vi "Configure.vi"(8 "error in (no error)":errorcluster) -> (0 "error out":errorcluster, 2 "groups":string[](array[string]), 3 "config":variant)   [LabVIEW 2017, in "DataAccumulator.lvlib"]
uses:
  <vilib>/addons/InsightCM/Devices/Shared/Common/DataAccumulator/DataAccumulator.lvlib
  <vilib>/addons/InsightCM/Devices/Shared/Common/DataAccumulator/controls/DataStoreOps.ctl
  <vilib>/addons/InsightCM/Devices/Shared/Common/DataAccumulator/controls/config.ctl
  <vilib>/addons/InsightCM/Devices/Shared/Common/DeviceHealth/controls/deviceHealthTag.ctl
  <vilib>/addons/InsightCM/Devices/Shared/Common/DeviceHealth/controls/SystemHealthTagEnum.ctl
  <vilib>/addons/InsightCM/MessageBus/Base/controls/Tag.ctl
  <vilib>/addons/InsightCM/MessageBus/Base/controls/KeyValuePair.ctl
  <vilib>/addons/InsightCM/Devices/Shared/Common/DataAccumulator/controls/AccumulationSettings.ctl
  <vilib>/addons/InsightCM/Devices/Shared/Common/DataAccumulator/controls/accumulationType.ctl
  <vilib>/addons/InsightCM/Devices/Shared/Common/DVRBuffer/controls/BufferLocation.ctl
  <vilib>/addons/InsightCM/Devices/Shared/Common/DVRBuffer/DVRBuffer.lvlib
  <vilib>/addons/InsightCM/Utilities/GlobalConfiguration/GlobalConfiguration.lvlib
  <vilib>/addons/InsightCM/Utilities/DeviceModelHelpers/DeviceModelHelpers.lvlib
  <vilib>/addons/InsightCM/Utilities/PropertyHelpers/PropertyHelpers.lvlib
  <vilib>/addons/InsightCM/Devices/Shared/Common/DeviceHealth/DeviceHealth.lvlib
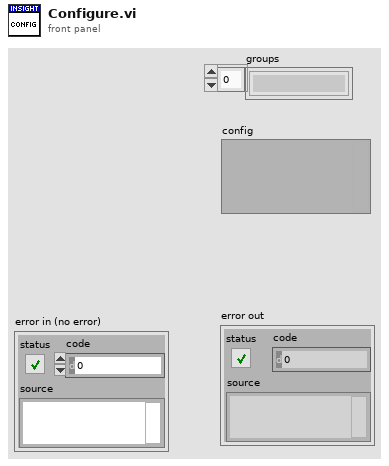
[diagram p1: front panel]
types:
  T1 = typedef "DataAccumulator.lvlib/DataStoreOps.ctl" = enum16{"Reset", "Init", "Clear", "SetWfms", "GetWfms"}
  T2 = typedef "SectionKeyValues.ctl" = cluster{"Section":string, "KeyValues":T3[]}
  T3 = typedef "KeyValuePair.ctl" = cluster{"Key":string, "Value":string}
  T4 = typedef "R2_DeviceModel.ctl" = cluster{"Device":T5, "Channels":T12[], "Tags":T14[]}
  T5 = typedef "R2_Device.ctl" = cluster{"Id":string, "Name":string, "DeviceType":string, "HardwareName":string, "IpAddress":string, "HardwareInfo":T3[], "ApplicationType":string, "ApplicationVersion":string, "EquipmentIds":string[], "ConfigurationVersion":string, "State":T6, "Properties":T3[], "DataGroups":T7[], "BurstModeTrigger":T11}
  T6 = typedef "DeviceState.ctl" = cluster{"Disabled":bool}
  T7 = typedef "R2_DataGroup.ctl" = cluster{"Name":string, "OperatingStates":T8[], "Properties":T3[], "EquipmentIds":string[], "AssetNodeId":string}
  T8 = typedef "OperatingState.ctl" = cluster{"Name":string, "Properties":T3[], "Triggers":T9[]}
  T9 = typedef "Trigger.ctl" = cluster{"Type":string, "Expression":string, "Conditions":T10[]}
  T10 = typedef "Condition.ctl" = cluster{"Source":string, "Type":string, "Operator":string, "CompareTo":string, "DwellSeconds":dbl}
  T11 = typedef "BurstModeTrigger.ctl" = cluster{"Trigger":T9, "SampleRate":string, "AcquisitionLength":string}
  T12 = typedef "R2_Channel.ctl" = cluster{"Id":string, "DeviceId":string, "Name":string, "ChannelType":string, "HardwareKey":string, "HardwareChannel":string, "DataGroup":string, "Keywords":string[], "EquipmentIds":string[], "Properties":T3[], "Metrics":T13[], "AssetNodeId":string, "MeasType":string, "AssetName":string}
  T13 = typedef "Metric.ctl" = cluster{"Id":string, "Name":string, "Unit":string, "Properties":T3[], "MetricDefinitionInstanceId":string}
  T14 = typedef "Tag.ctl" = cluster{"Id":string, "Path":string, "Name":string, "Datatype":string, "Props":T3[], "Keywords":string[]}
  T15 = typedef "DataAccumulator.lvlib/config.ctl" = cluster{"Group":string, "BlockComplete":bool, "Ok To Start":bool, "Speed Ref Chan":string, "Current OpState":string, "MaxLowRateCPU(%)":dbl, "MaxLowRateMem(%)":dbl, "LowRateCount":i32, "LowRateCountTag":T16}
  T16 = typedef "DeviceHealth.lvlib/deviceHealthTag.ctl" = cluster{"SystemTags":T17, "TagId":string, "Tag":T14}
  T17 = typedef "DeviceHealth.lvlib/SystemHealthTagEnum.ctl" = enum16{"CPU Utilization", "Memory Utilization", "Disk Utilization", "Total Physical Memory", "Primary Disk Free", "Chassis Temperature", "LowRateCount"}
  T18 = typedef "DataAccumulator.lvlib/AccumulationSettings.ctl" = cluster{"Type":T19, "Length":dbl, "Max Time (sec)":dbl, "Start Block":T20, "Acquired (sec)":dbl, "Acquired (pulses)":i32, "Initial Pulse Offset":dbl, "Stop Block":T20, "LastBlockAdded":u32}
  T19 = typedef "DataAccumulator.lvlib/accumulationType.ctl" = enum16{"none", "seconds", "revolutions"}
  T20 = typedef "DVRBuffer.lvlib/BufferLocation.ctl" = cluster{"Block":u32, "Index":i32}
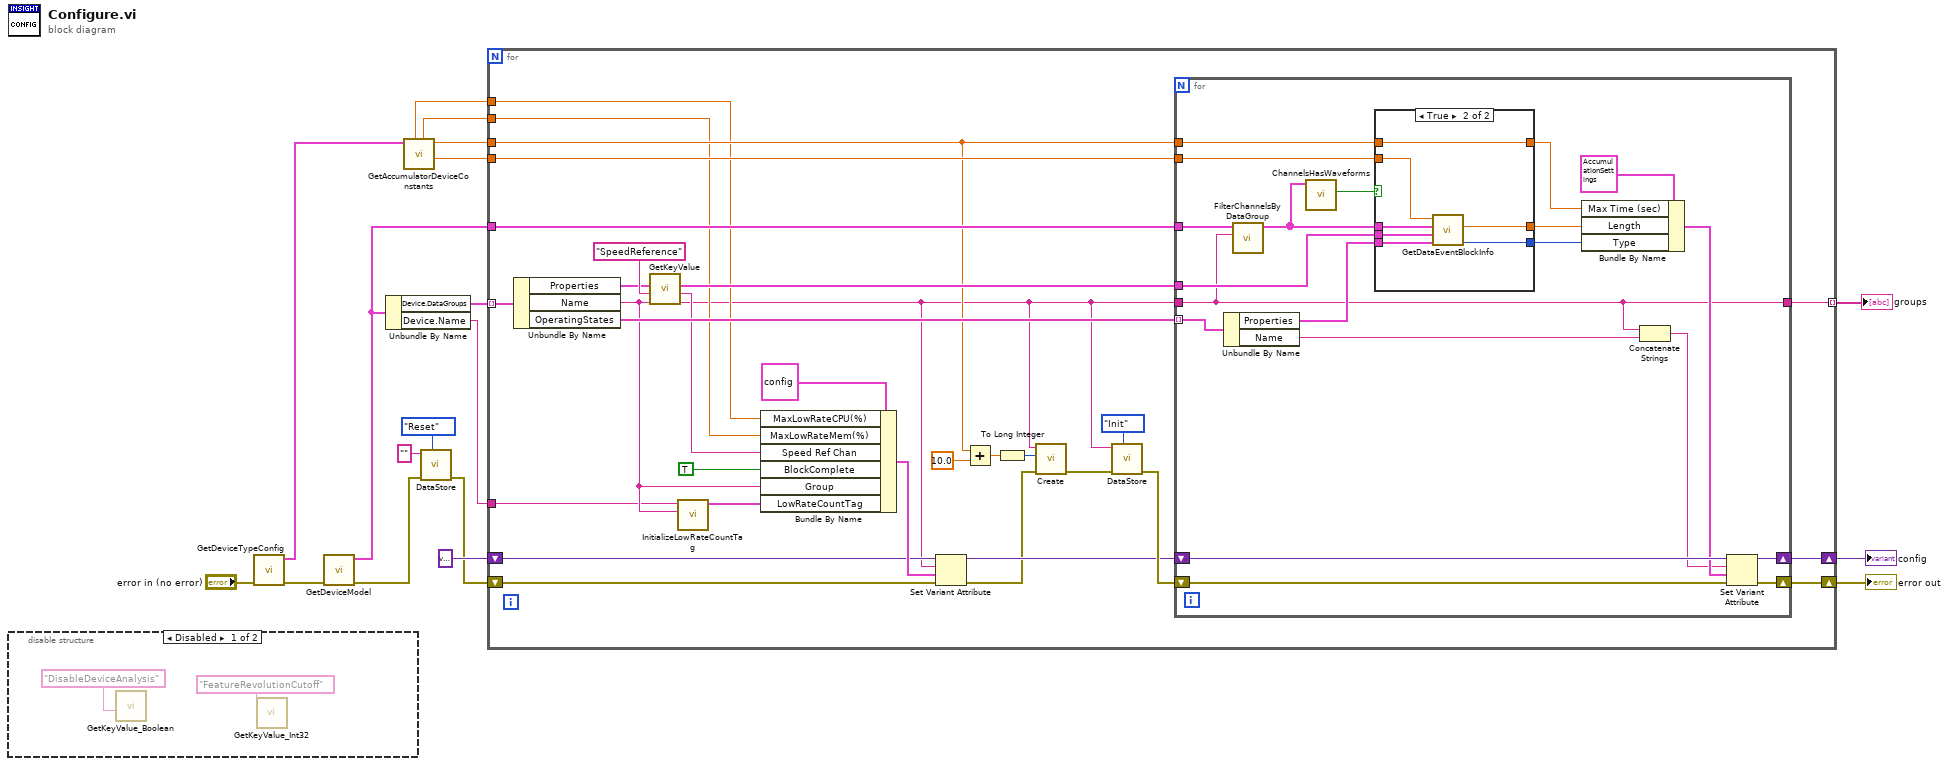
[diagram p0: block diagram]
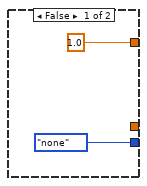
[diagram p3: hidden frame]
diagram:
  n1 = disable-structure shown="Disabled" {
    frame Disabled {
      n2 = call <vilib>:"GetKeyValue_Boolean.vi"("key"="DisableDeviceAnalysis") -> ()  [unwired: 8 in, 3 out]
      n3 = call <vilib>:"GetKeyValue_Int32.vi"("key"="FeatureRevolutionCutoff") -> ()  [unwired: 8 in, 3 out]
    }
    frame Enabled {
    }
  }
  n4 = call <vilib>:"GetDeviceTypeConfig.vi"("error in (no error)"="error in (no error)") -> ("error out"=w11:errorcluster, "key values"=w13:T2[])  [unwired: 8 in, 1 out]
  n5 = call <vilib>:"GetDeviceModel.vi"("error in (no error)"=w11) -> ("error out"=w2:errorcluster, "device model"=w14:T4)  [unwired: 8 in, 1 out]
  n6 = Unbundle By Name(w14) -> ("Device.DataGroups"=w18:T7[], "Device.Name"=w6:string)
  n7 = call <vilib>:"GetAccumulatorDeviceConstants.vi"("key values"=w13) -> ("default data block length (sec)"=w10:dbl, "max block (sec)"=w9:dbl, "max low rate memory (percent)"=w8:dbl, "max low rate cpu (percent)"=w7:dbl)  [unwired: 6 in, 1 out]
  n8 = call <vilib>:"DataStore.vi"("operation"=DataStoreOps."Reset", "error in (no error)"=w2, "group"="") -> ("error out"=w1:errorcluster)  [unwired: 7 in, 1 out]
  n9 = for {
    tunnel: w18 -> [w49] mode=indexing
    shift-right: [w50] -> w17
    shift-left: variant -> [w30]
    shift-right: [w41] -> w15
    shift-left: w1 -> [w28]
    tunnel: w14 -> [w48]
    tunnel: w9 -> [w37]
    tunnel: w10 -> [w47]
    tunnel: w8 -> [w26]
    tunnel: w7 -> [w25]
    tunnel: w6 -> [w22]
    tunnel: [w21] -> w5 mode=indexing
    n10 = Unbundle By Name(w49) -> ("Properties"=w39:T3[], "Name"=w23:string, "OperatingStates"=w45:T8[])
    n11 = call <vilib>:"GetKeyValue.vi"("key"="SpeedReference", "key value pairs"=w39) -> ("value"=w33:string, "key value pairs out"=w38:T3[])  [unwired: 7 in, 1 out]
    n12 = call <vilib>:"InitializeLowRateCountTag.vi"("Group"=w23, "Device"=w22) -> ("LowRateCountTag"=w24:T16)  [unwired: 9 in]
    n13 = Bundle By Name(cluster=T15 {"Group"="", "BlockComplete"=FALSE, "Ok To Start"=FALSE, "Speed Ref Chan"="", "Current OpState"="", "MaxLowRateCPU(%)"=0.0, "MaxLowRateMem(%)"=0.0, "LowRateCount"=0, "LowRateCountTag"={"SystemTags"=enum."CPU Utilization", "TagId"="", "Tag"={"Id"="", "Path"="", "Name"="", "Datatype"="", "Props"=[], "Keywords"=[]}}} ("Config"), "MaxLowRateCPU(%)"=w25, "MaxLowRateMem(%)"=w26, "Speed Ref Chan"=w33, "BlockComplete"=TRUE ("OkToStart"), "Group"=w23, "LowRateCountTag"=w24) -> (w35:T15)
    n14 = Set Variant Attribute(Variant=w30, name=w23, value=w35, error in=w28) -> (Variant out=w29:variant, error out=w27:errorcluster)  [unwired: 1 out]
    n15 = Add(x=w37, y=10.0) -> (x+y=w44:dbl)
    n16 = To Long Integer(number=w44) -> (32bit integer=w43:i32)
    n17 = call <vilib>:"Create.vi"("error in (no error)"=w27, "size"=w43, "name"=w23) -> ("error out"=w32:errorcluster)  [unwired: 7 in, 1 out]
    n18 = call <vilib>:"DataStore.vi"("operation"=DataStoreOps."Init", "error in (no error)"=w32, "group"=w23) -> ("error out"=w31:errorcluster)  [unwired: 7 in, 1 out]
    n19 = for {
      tunnel: w48 -> [w64]
      tunnel: w47 -> [w62]
      tunnel: w37 -> [w61]
      tunnel: w23 -> [w51]
      tunnel: w38 -> [w58]
      shift-right: [w68] -> w50
      shift-left: w29 -> [w70]
      shift-right: [w60] -> w41
      shift-left: w31 -> [w69]
      tunnel: w45 -> [w57] mode=indexing
      tunnel: [w51] -> w21
      n20 = Unbundle By Name(w57) -> ("Properties"=w56:T3[], "Name"=w54:string)
      n21 = call <vilib>:"FilterChannelsByDataGroup.vi"("group"=w51, "device model"=w64) -> ("channels in data group"=w63:T12[])  [unwired: 8 in, 1 out]
      n22 = call <vilib>:"ChannelsHasWaveforms.vi"("channels"=w63) -> ("has waveforms"=w59:bool)  [unwired: 10 in]
      n23 = case shown="True" w59 {
        tunnel: [accumulationType."none" ("type") w78] -> w66
        tunnel: [_ w77] -> w65
        tunnel: w63 -> [_ w74]
        tunnel: w62 -> [_ w73]
        tunnel: [1.0 ("max block (sec)") w79] -> w55
        tunnel: w61 -> [_ w79]
        tunnel: w58 -> [_ w75]
        tunnel: w56 -> [_ w76]
        frame False {
        }
        frame True {
          n24 = call <vilib>:"GetDataEventBlockInfo.vi"("operating state properties"=w76, "group properties"=w75, "channels"=w74, "default data block length"=w73) -> ("type"=w78:T19, "total length"=w77:dbl)  [unwired: 2 in, 4 out]
        }
      }
      n25 = Bundle By Name(cluster=T18 {"Type"=enum."none", "Length"=0.0, "Max Time (sec)"=0.0, "Start Block"={"Block"=0, "Index"=0}, "Acquired (sec)"=0.0, "Acquired (pulses)"=0, "Initial Pulse Offset"=0.0, "Stop Block"={"Block"=0, "Index"=0}, "LastBlockAdded"=0} ("Accumulation Settings"), "Max Time (sec)"=w55, "Length"=w65, "Type"=w66) -> (w67:T18)
      n26 = Concatenate Strings(w51, w54) -> (w53:string)
      n27 = Set Variant Attribute(Variant=w70, name=w53, value=w67, error in=w69) -> (Variant out=w68:variant, error out=w60:errorcluster)  [unwired: 1 out]
    }
  }
  "config" <- w17
  "error out" <- w15
  "groups" <- w5
